vi "Merc test.vi"() -> ()   [LabVIEW 2015]
panel:
  out "Magnetic Field (T)":dbl
  in  "VISA resource name":refnum<visa-resource-name>
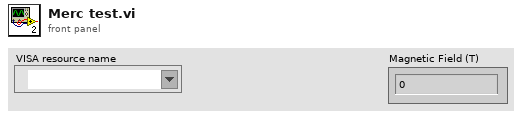
[diagram p1: front panel]
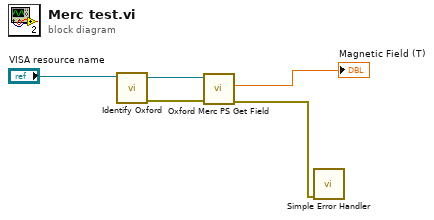
[diagram p0: block diagram]
diagram:
  n1 = call "Identify Oxford.vi"("VISA resource name"="VISA resource name") -> ("error out"=w4:errorcluster, "VISA resource name out"=w3:refnum<visa-resource-name>)  [unwired: 6 in, 3 out]
  n2 = call "Oxford Merc PS Get Field.vi"("Error In"=w4, "VISA resource name"=w3) -> ("Error Out"=w1:errorcluster, "Magnetic Field (T)"=→"Magnetic Field (T)":dbl)  [unwired: 7 in, 1 out]
  n3 = call <vilib>:"Simple Error Handler.vi"("error in (no error)"=w1) -> ()  [unwired: 4 in, 5 out]
